vi "FaulhaberV3Read.vi"(8 "error in (no error)":errorcluster, 11 "VISA Refnum in":refnum<visa-resource-name>) -> (0 "error out":errorcluster, 1 "Value":u8[](array[numeric]) format="%02x", 2 "Object":u32 format="%08x", 3 "VISA Refnum out":refnum<visa-resource-name>, 5 "unsigned byte array":u8[](array[numeric]) format="%02x")   [LabVIEW 2011]
uses:
  <vilib>/Instr/_visa.llb/VISA Flush IO Buffer Mask.ctl
panel:
  out "Return is":T1(ring)=enum."SDORead"
  out "Axis":u8
  out "return count":u32=6
  # "string? hier nicht in Zahl wandeln?"
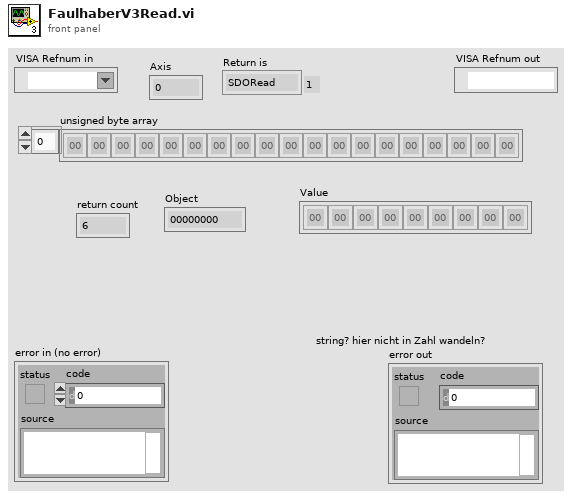
[diagram p1: front panel]
types:
  T1 = enum8{"Bootup", "SDORead", "SDOWrite", "SDOErrror", "Controlword", "Statusword", "TraceLog", "Emcy", "SDOBlockReadInit", "SDOBlockReadUpload", "SDOBlockReadEnd", "SDOBlockWriteInit", "SDOBlockWriteDownload", "SDOBlockWriteEnd"}
  T2 = typedef "VISA Flush IO Buffer Mask.ctl" = u16
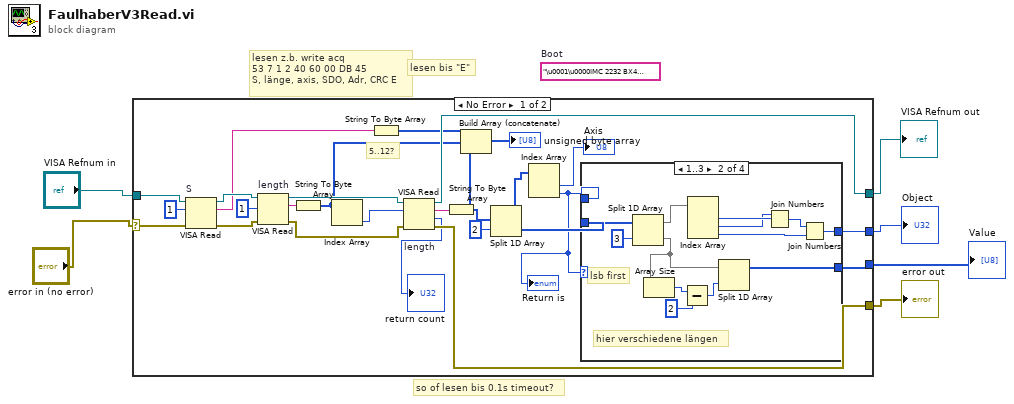
[diagram p0: block diagram]
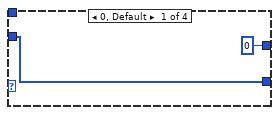
[diagram p2: hidden frame]
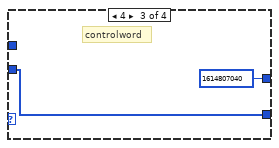
[diagram p3: hidden frame]
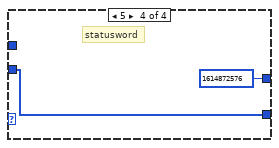
[diagram p4: hidden frame]
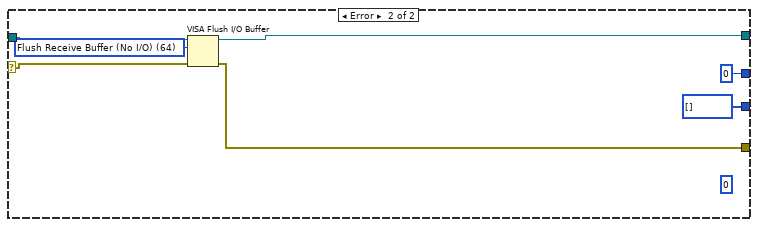
[diagram p5: hidden frame]
diagram:
  (unwired) "\u0001\u0000IMC 2232 BX4 RS¤E"  # Boot
  # "so of lesen bis 0.1s timeout?"
  # "lesen bis \"E\""
  # "lesen z.b. write acq\n53 7 1 2 40 60 00 DB 45\nS, länge, axis, SDO, Adr, CRC E"
  n1 = case shown="No Error" "error in (no error)" {
    selector: "error in (no error)" -> [w30 w56]
    tunnel: "VISA Refnum in" -> [w31 w58]
    tunnel: [w20 w57] -> w5
    tunnel: [w22 w55] -> w6
    tunnel: [w15 u32 0] -> w2
    tunnel: [w14 u8[] []] -> w1
    frame No Error {
      # "5..12?"
      n2 = VISA Read "S"(VISA resource name=w31, byte count=u32 1, error in (no error)=w30) -> (VISA resource name out=w28:refnum<visa-resource-name>, read buffer=w8:string, error out=w29:errorcluster)  [unwired: 1 out]
      n3 = VISA Read "length"(VISA resource name=w28, byte count=u32 1, error in (no error)=w29) -> (VISA resource name out=w26:refnum<visa-resource-name>, read buffer=w25:string, error out=w23:errorcluster)  [unwired: 1 out]
      n4 = String To Byte Array(string=w25) -> (unsigned byte array=w9:u8[])
      n5 = Index Array(array=w9) -> (element=w24:u8)  [unwired: 1 in]
      n6 = String To Byte Array(string=w8) -> (unsigned byte array=w7:u8[])
      n7 = VISA Read "length"(VISA resource name=w26, byte count=w24, error in (no error)=w23) -> (VISA resource name out=w20:refnum<visa-resource-name>, read buffer=w21:string, return count=→"return count":u32, error out=w22:errorcluster)
      n8 = String To Byte Array(string=w21) -> (unsigned byte array=w18:u8[])
      n9 = Build Array (concatenate)(w7, w9, w18) -> (→"unsigned byte array":u8[])
      n10 = Split 1D Array(array=w18, index=2) -> (first subarray=w13:u8[], second subarray=w16:u8[])
      n11 = Index Array(array=w13) -> (element #1=→"Axis":u8, element #2=w11:u8)  [unwired: 2 in]
      "Return is" <- w11
      n12 = case shown="1..3" w11 {
        tunnel: w16 -> [w34 w43 w49 w51]
        tunnel: [u32 0 w36 u32 1614807040 u32 1614872576] -> w15
        tunnel: [w34 w35 w49 w51] -> w14
        tunnel: w11 -> [_ _ _ _]
        frame 0, Default {
        }
        frame 1..3 {
          # "lsb first"
          # "hier verschiedene längen"
          n13 = Split 1D Array(array=w43, index=3) -> (first subarray=w41:u8[], second subarray=w40:u8[])
          n14 = Array Size(array=w40) -> (size(s)=w39:i32)
          n15 = Subtract(x=w39, y=2) -> (x-y=w37:i32)
          n16 = Index Array(array=w41) -> (element #1=w47:u8, element #2=w46:u8, element #3=w44:u8)  [unwired: 3 in]
          n17 = Split 1D Array(array=w40, index=w37) -> (first subarray=w35:u8[])  [unwired: 1 out]
          n18 = Join Numbers(hi=w46, lo=w47) -> ((hi.lo)=w45:u16)
          n19 = Join Numbers(hi=w45, lo=w44) -> ((hi.lo)=w36:u32)
        }
        frame 4 {
          # "controlword"
        }
        frame 5 {
          # "statusword"
        }
      }
    }
    frame Error {
      (unwired) 0
      w54 = T2 64 items=["Flush Receive Buffer"=16, "Write Transmit Buffer to Device"=32, "Flush Receive Buffer (No I/O)"=64, "Flush Transmit Buffer"=128] ("Mask")
      n20 = VISA Flush I/O Buffer(VISA resource name=w58, mask (16)=w54, error in (no error)=w56) -> (VISA resource name out=w57:refnum<visa-resource-name>, error out=w55:errorcluster)
    }
  }
  "error out" <- w6
  "Object" <- w2
  "VISA Refnum out" <- w5
  "Value" <- w1
